vi "PTScanner.get step obj params.vi"(1 "Objects":T1[](array[typedef]), 4 "step object params":T3) -> (5 "obj index":i32, 6 "Minus Delta":dbl, 7 "obj params":T1, 8 "Plus Delta":dbl, 9 "nomValue":dbl, 10 "increment":dbl, 11 "range":dbl, 12 "Centroid":dbl, 13 "actValue":dbl, 14 "Object":string, 15 "DIM Service Address":string, 16 "Set value method":string, 17 "Data descriptor":string, 18 "Method Input Parameters":T2(array[cluster]), 19 "Call Mode":enum16{"Simple DIM", "Synchronous"}(ring))   [LabVIEW 2014, in "PTScanner.lvlib"]
uses:
  PTScanner.lvlib
  PTScanner.obj parameters.ctl
  PTScanner.step obj parameters.ctl
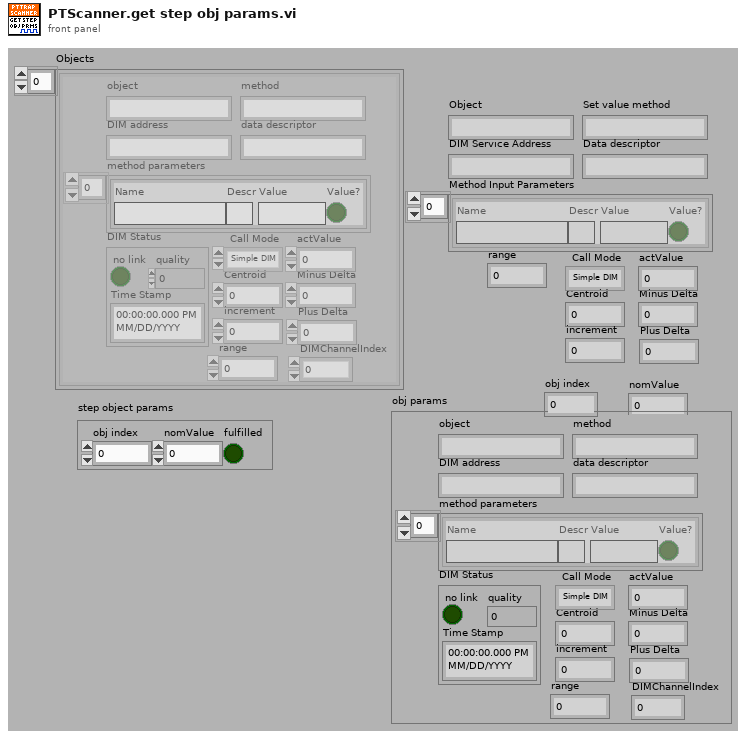
[diagram p1: front panel]
types:
  T1 = typedef "PTScanner.lvlib/PTScanner.obj parameters.ctl" = cluster{"object":string, "DIM address":string, "method":string, "data descriptor":string, "method parameters":cluster{"Name":string, "Descr":string, "Value":string, "Value?":bool}[], "Call Mode":enum16{"Simple DIM", "Synchronous"}, "actValue":dbl, "Centroid":dbl, "Minus Delta":dbl, "Plus Delta":dbl, "increment":dbl, "DIM Status":cluster{"no link":bool, "quality":i32, "Time Stamp":timestamp}, "range":dbl, "DIMChannelIndex":i32}
  T2 = cluster{"Name":string, "Descr":string, "Value":string, "Value?":bool}[]
  T3 = typedef "PTScanner.lvlib/PTScanner.step obj parameters.ctl" = cluster{"obj index":i32, "nomValue":dbl, "fulfilled":bool}
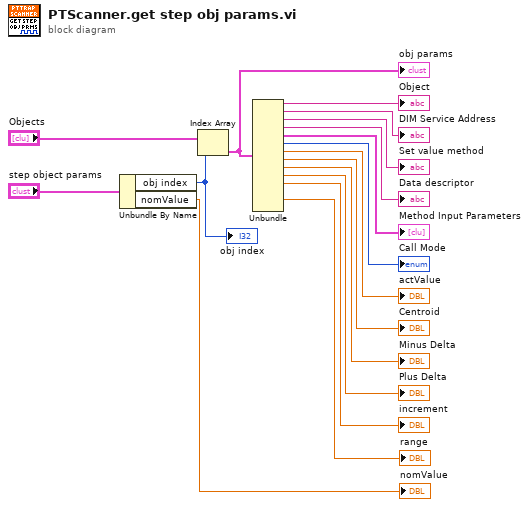
[diagram p0: block diagram]
diagram:
  n1 = Unbundle By Name("step object params") -> ("obj index"=w15:i32, "nomValue"=→"nomValue":dbl)
  "obj index" <- w15
  n2 = Index Array(array="Objects", index=w15) -> (element=w4:T1)
  "obj params" <- w4
  n3 = Unbundle(w4) -> ("object"=→"Object":string, "DIM address"=→"DIM Service Address":string, "method"=→"Set value method":string, "data descriptor"=→"Data descriptor":string, "method parameters"=→"Method Input Parameters":T2, "Call Mode"=→"Call Mode":enum16{"Simple DIM", "Synchronous"}, "actValue"=→"actValue":dbl, "Centroid"=→"Centroid":dbl, "Minus Delta"=→"Minus Delta":dbl, "Plus Delta"=→"Plus Delta":dbl, "increment"=→"increment":dbl, "range"=→"range":dbl)  [unwired: 2 out]
